vi "parallel move.vi"   [LabVIEW 2016, in "Test.lvrbt"]
uses:
  Test.lvrbt
  <vilib>/NXT/Hardware/Plugins/Tetrix DC Motor/TetrixDCMotorAddress.ctl
  <vilib>/NXT/NXTIO Xnodes/NXTIONodeSubVIs/TETRIX IO Move DC Motors.vi
  <vilib>/NXT/Dual Mode Library/Waits/Wait_Num(msec).vi
  <vilib>/NXT/NXTIO Xnodes/NXTIONodeSubVIs/LEGOStopAllMotors.vi
  <vilib>/NXT/NXTIO Xnodes/NXTIONodeSubVIs/TETRIX IO Stop DC Motors.vi
  <vilib>/NXT/NXTIO Xnodes/AddressXNode/NXTIOAddress.xnode
  <vilib>/NXT/Subs/LVHSConnector.ctl
  <vilib>/NXT/NXTIO Xnodes/NXTIOXNode/NXTIO.xnode
  <vilib>/NXT/LegoClasses/BrickReference/BrickReference.lvclass
types:
  T1 = typedef "TetrixDCMotorAddress.ctl" = i32
  T2 = typedef "LVHSConnector.ctl" = refnum<class "BrickReference.lvclass">
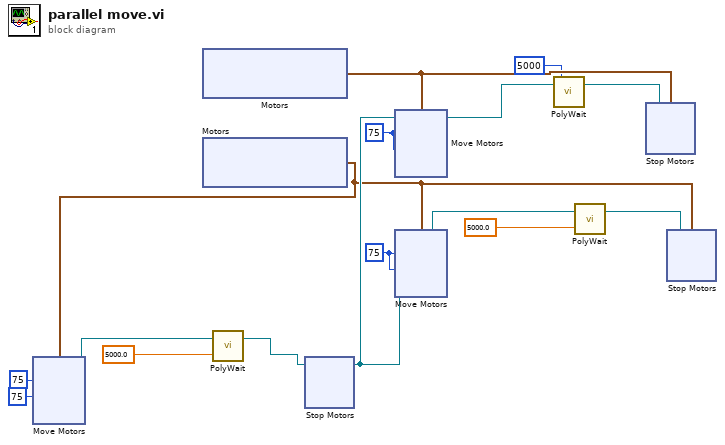
[diagram p0: block diagram]
diagram:
  w9 = i8 75 ("Power/Speed 1")
  w13 = i8 75 ("Power/Speed 1")
  n1 = xnode "Motors"() -> ("Motor"=w11:cluster{"TetrixDCMotor":T1, "TetrixDCMotor":T1})
  n2 = xnode "Motors"() -> ("Motor"=w2:cluster{"TetrixDCMotor":T1, "TetrixDCMotor":T1})
  n3 = xnode "Move Motors"("Power/Speed 2"=i8 75, "Power/Speed 1"=i8 75, "Motors"=w2) -> ("NXT/EV3"=w5:T2)  [unwired: 1 in]
  n4 = call-poly <vilib>:"PolyWait.vi"("Time (100 msec)"=sgl 5000.0 ("Time (1 sec)"), "NXT/EV3"=w5) -> ("NXT/EV3"=w4:T2)  [unwired: 2 in]
  n5 = xnode "Stop Motors"("NXT/EV3"=w4) -> ("NXT/EV3"=w3:T2)  [unwired: 1 in]
  n6 = xnode "Move Motors"("Power/Speed 2"=w9, "Power/Speed 1"=w9, "Motors"=w11, "NXT/EV3"=w3) -> ("NXT/EV3"=w10:T2)
  n7 = xnode "Move Motors"("Power/Speed 2"=w13, "Power/Speed 1"=w13, "Motors"=w2, "NXT/EV3"=w3) -> ("NXT/EV3"=w16:T2)
  n8 = call-poly <vilib>:"PolyWait.vi"("Time (100 msec)"=u32 5000, "NXT/EV3"=w10) -> ("NXT/EV3"=w12:T2)  [unwired: 2 in]
  n9 = call-poly <vilib>:"PolyWait.vi"("Time (100 msec)"=sgl 5000.0 ("Time (1 sec)"), "NXT/EV3"=w16) -> ("NXT/EV3"=w14:T2)  [unwired: 2 in]
  n10 = xnode "Stop Motors"("Motors"=w11, "NXT/EV3"=w12) -> ()  [unwired: 1 out]
  n11 = xnode "Stop Motors"("Motors"=w2, "NXT/EV3"=w14) -> ()  [unwired: 1 out]
